vi "EMV T6 T7 Flow Detect.vi"(0 "T7 Detect?":bool, 1 "User Setpoint Temperature":u16=125, 3 "Mixing Valve.T6 Temp (0x406E)":dbl, 5 "T6_OFFSET_FROM_TARGET_INDICATING_FLOW":dbl=3.0, 7 "T6_DELTA_INDICATING_FLOW":dbl=2.0, 11 "error in (no error)":errorcluster) -> (4 "Flow Dectection":bool, 15 "error out":errorcluster)   [LabVIEW 2016]
panel:
  # "T6 Data"
  # "Basic Inputs"
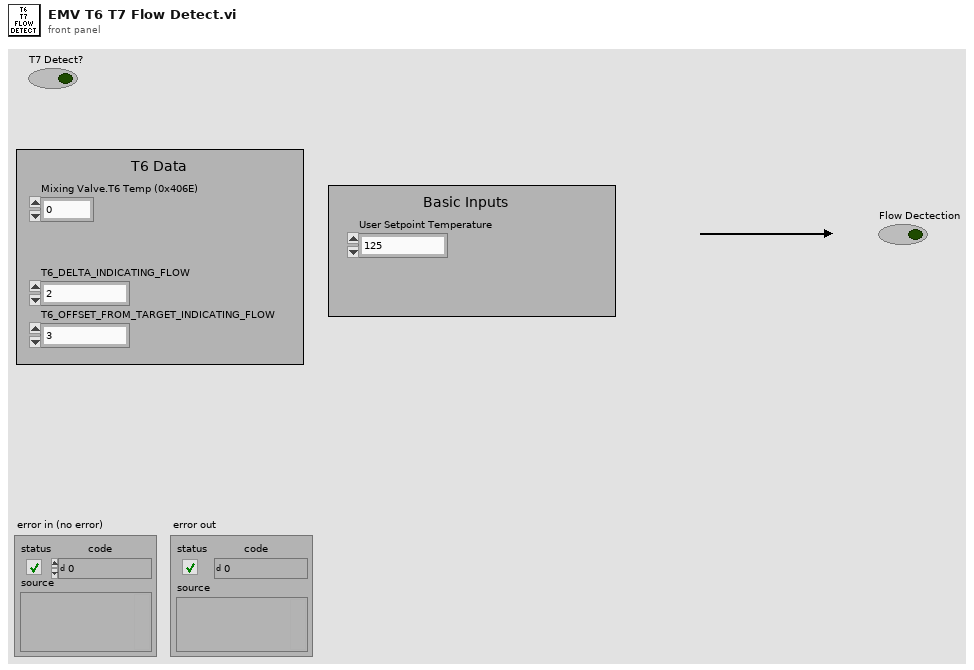
[diagram p1: front panel]
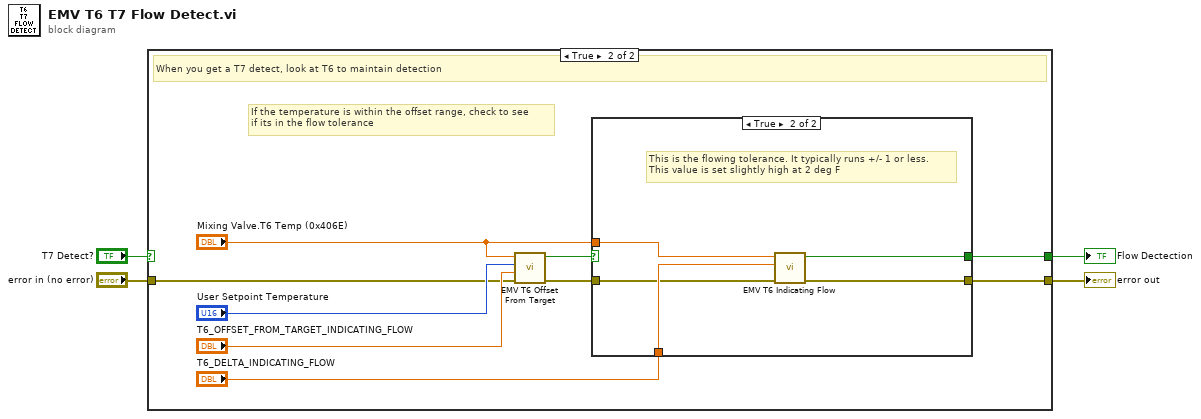
[diagram p0: block diagram]
diagram:
  n1 = case shown="True" "T7 Detect?" {
    selector: "T7 Detect?" -> [w6 _]
    tunnel: [w6 w7] -> w4
    tunnel: "error in (no error)" -> [w5 w13]
    tunnel: [w5 w9] -> w1
    frame False {
      # "If no T7 detect...do nothing"
    }
    frame True {
      # "If the temperature is within the offset range, check to see \nif its in the flow tolerance"
      # "When you get a T7 detect, look at T6 to maintain detection"
      n2 = call "EMV T6 Offset From Target.vi"("error in (no error)"=w13, "T6_OFFSET_FROM_TARGET_INDICATING_FLOW"="T6_OFFSET_FROM_TARGET_INDICATING_FLOW", "User Setpoint Temperature"="User Setpoint Temperature", "Mixing Valve.T6 Temp (0x406E) in"="Mixing Valve.T6 Temp (0x406E)") -> ("error out"=w10:errorcluster, "Flow Dectection"=w8:bool)  [unwired: 6 in]
      n3 = case shown="True" w8 {
        selector: w8 -> [w17 _]
        tunnel: "Mixing Valve.T6 Temp (0x406E)" -> [_ w22]
        tunnel: "T6_DELTA_INDICATING_FLOW" -> [_ w21]
        tunnel: w10 -> [w16 w20]
        tunnel: [w16 w19] -> w9
        tunnel: [w17 w18] -> w7
        frame False {
        }
        frame True {
          # "This is the flowing tolerance. It typically runs +/- 1 or less. \nThis value is set slightly high at 2 deg F"
          # "If the temperature is within the offset range, check to see it i"
          n4 = call "EMV T6 Indicating Flow.vi"("error in (no error)"=w20, "T6_DELTA_INDICATING_FLOW"=w21, "Mixing Valve.T6 Temp (0x406E)"=w22) -> ("error out"=w19:errorcluster, "Flow Dectection"=w18:bool)  [unwired: 7 in]
        }
      }
    }
  }
  "Flow Dectection" <- w4
  "error out" <- w1
